vi "BRig_dataCurrent_DAB_HighProb.vi"() -> (2 "output_DAB_HighProb":i32)   [LabVIEW 2014]
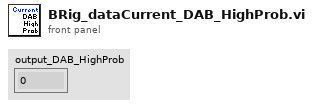
[diagram p1: front panel]
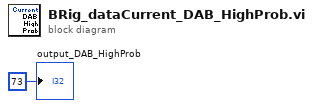
[diagram p0: block diagram]
diagram:
  "output_DAB_HighProb" <- 73 ("output_iBlock")
